vi "ReadRackControllerParameters(BothRacks).vi"(8 "error in":errorcluster, 9 "Part Name":string, 10 "JSON file path":path=path "C:/Users/raakeshs/Desktop/ppts/JSON/Write to JSON String/data/Files/test4.json", 11 "Input ListBox Cluster":T1) -> (0 "error out":errorcluster, 3 "output cluster":T1)   [LabVIEW 2015]
uses:
  ZenGage v3.0 UI.lvclass
  Type Definitions/Edit tolerance settings/Rack Selection.ctl
  Type Definitions/Edit tolerance settings/Edit Tolerance Input.ctl
  <vilib>/Utility/miscctls.llb/LVPoint32TypeDef.ctl
  Type Definitions/Edit tolerance settings/ETL controls.ctl
panel:
  in  "Rack Number":i32
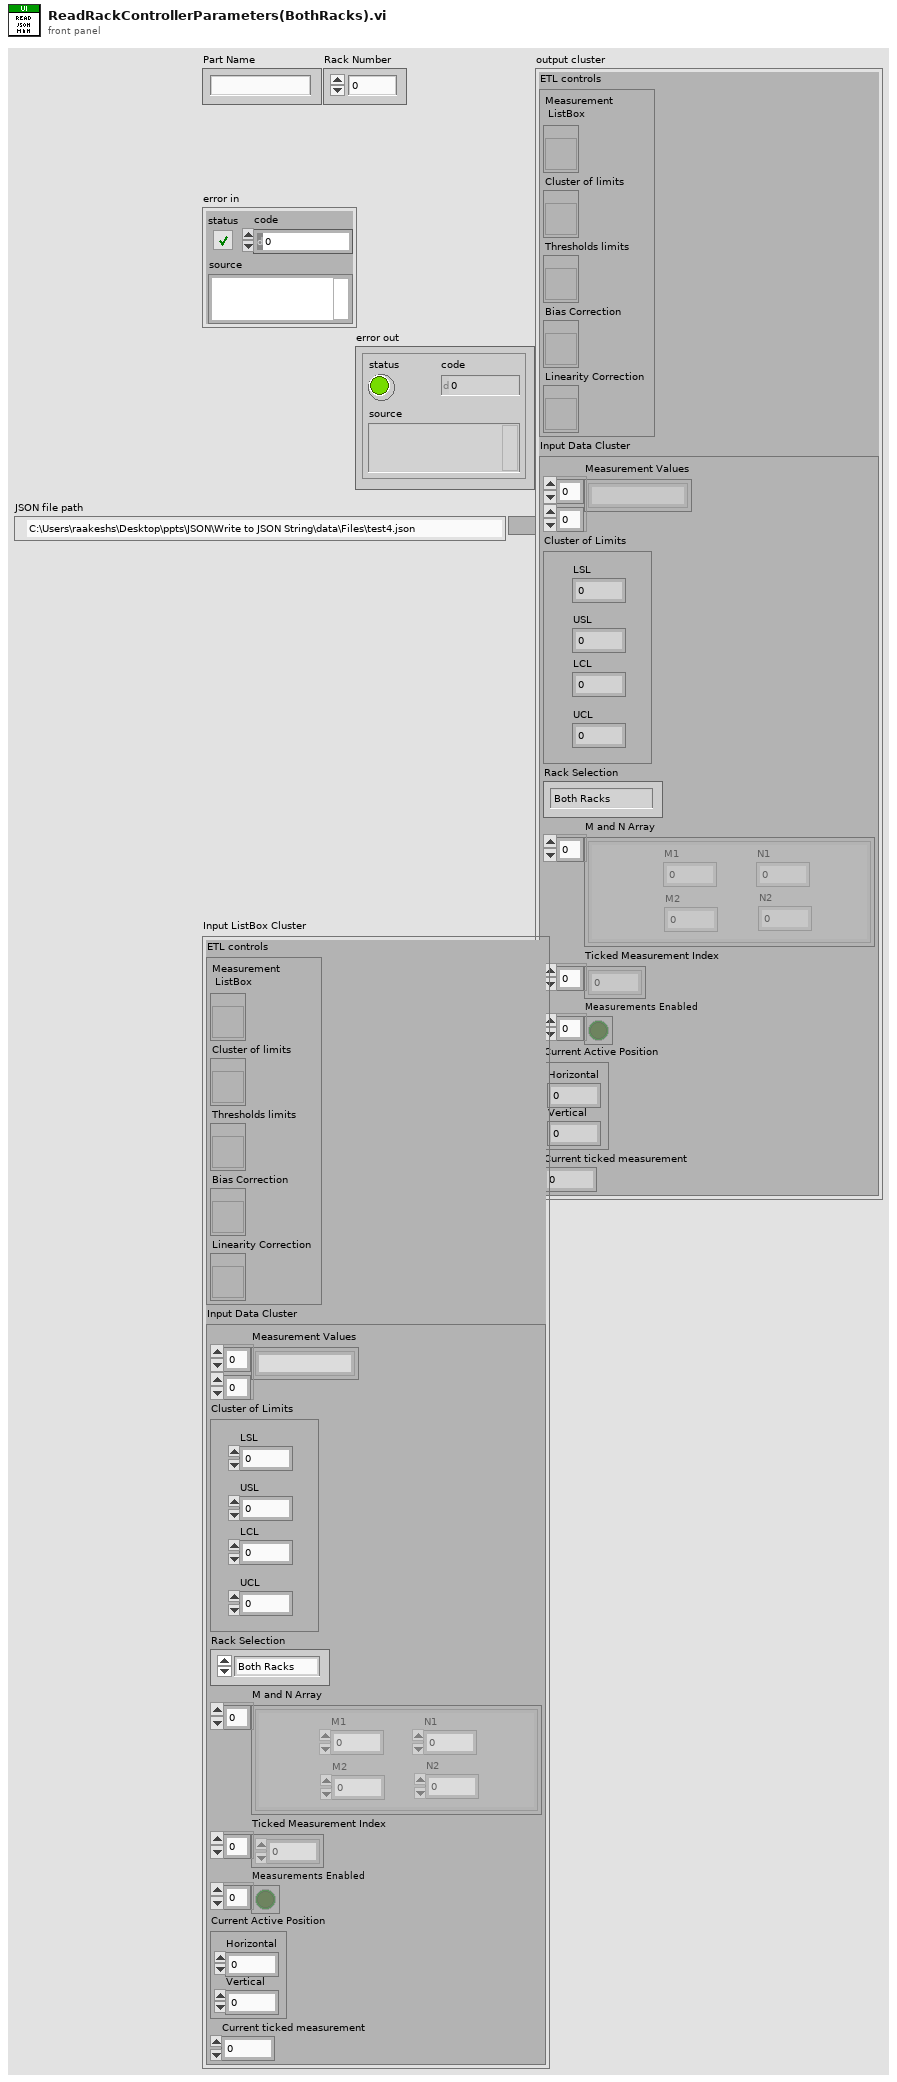
[diagram p1: front panel]
types:
  T1 = typedef "ZenGage v3.0 UI.lvclass/Edit Tolerance Input.ctl" = cluster{"ETL controls":T2, "Input Data Cluster":cluster{"Measurement Values":string[][], "Cluster of Limits":cluster{"LSL":dbl, "USL":dbl, "LCL":dbl, "UCL":dbl}, "Rack Selection":T3, "M and N Array":cluster{"M1":u64, "M2":u64, "N1":u64, "N2":u64}[], "Ticked Measurement Index":u32[], "Measurements Enabled":bool[], "Current Active Position":T4, "Current ticked measurement":dbl}}
  T2 = typedef "ETL controls.ctl" = cluster{"Measurement\n ListBox":refnum<vi>, "Cluster of limits":refnum<vi>, "Thresholds limits":refnum<vi>, "Bias Correction":refnum<vi>, "Linearity Correction":refnum<vi>}
  T3 = typedef "ZenGage v3.0 UI.lvclass/Rack Selection.ctl" = enum16{"Both Racks", "Rack 2", "Rack 1"}
  T4 = typedef "LVPoint32TypeDef.ctl" = cluster{"Horizontal":i32, "Vertical":i32}
  T5 = cluster{"RackControllerParameters":cluster{"RackId":i32, "PartsList":cluster{"Name":string, "ControlLimitsViolationThreshold":cluster{"M1":u64, "N1":u64}, "SpecificationLimitViolationThreshold":cluster{"M2":u64, "N2":u64}}[]}[]}
  T6 = cluster{"RackId":i32, "PartsList":cluster{"Name":string, "ControlLimitsViolationThreshold":cluster{"M1":u64, "N1":u64}, "SpecificationLimitViolationThreshold":cluster{"M2":u64, "N2":u64}}[]}[]
  T7 = cluster{"RackId":i32, "PartsList":cluster{"Name":string, "ControlLimitsViolationThreshold":cluster{"M1":u64, "N1":u64}, "SpecificationLimitViolationThreshold":cluster{"M2":u64, "N2":u64}}[]}
  T8 = cluster{"Name":string, "ControlLimitsViolationThreshold":cluster{"M1":u64, "N1":u64}, "SpecificationLimitViolationThreshold":cluster{"M2":u64, "N2":u64}}[]
  T9 = cluster{"Name":string, "ControlLimitsViolationThreshold":cluster{"M1":u64, "N1":u64}, "SpecificationLimitViolationThreshold":cluster{"M2":u64, "N2":u64}}
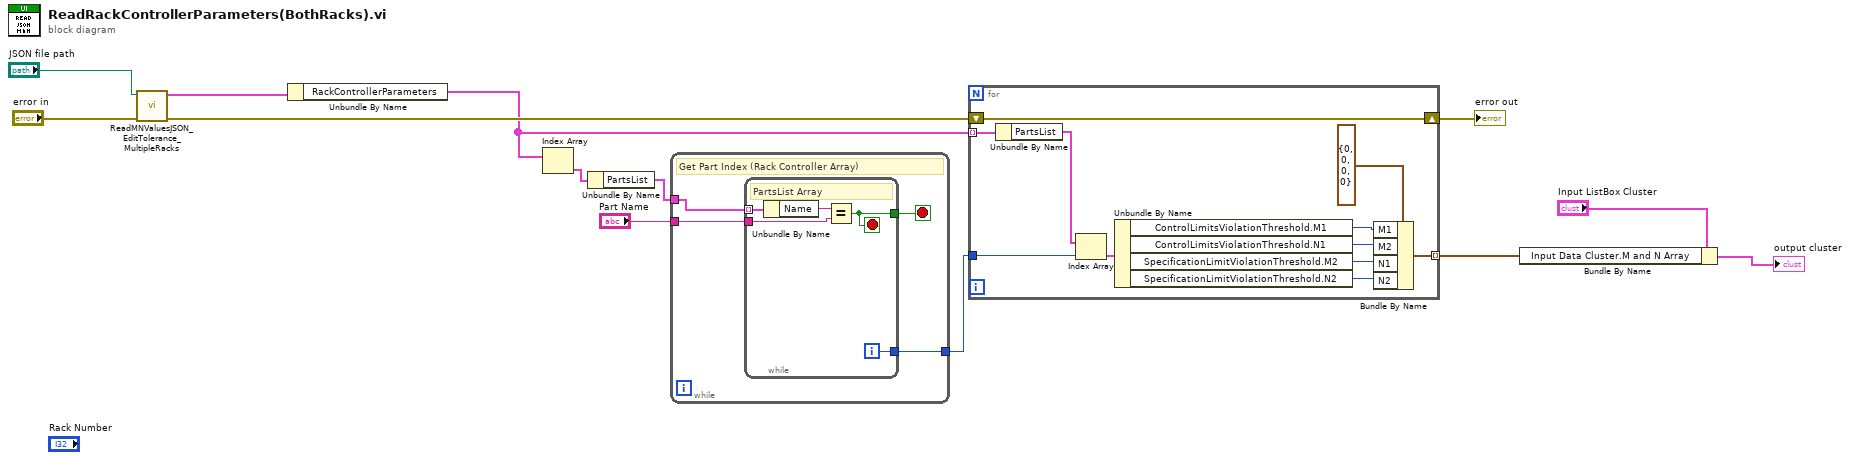
[diagram p0: block diagram]
diagram:
  n1 = call "ReadMNValuesJSON_EditTolerance_MultipleRacks.vi"("error in"="error in", "JSON file path"="JSON file path") -> ("error out"=w10:errorcluster, "Rack Controller Parameters out"=w12:T5)  [unwired: 8 in]
  n2 = Unbundle By Name(w12) -> ("RackControllerParameters"=w7:T6)
  n3 = Index Array(array=w7) -> (element=w2:T7)  [unwired: 1 in]
  n4 = Unbundle By Name(w2) -> ("PartsList"=w1:T8)
  n5 = while {
    tunnel: "Part Name" -> [w17]
    tunnel: [w15] -> w6
    tunnel: w1 -> [w14]
    stop <- w16 stop-if-true
    # "Get Part Index (Rack Controller Array)"
    n6 = while {
      tunnel: w14 -> [w22] mode=indexing
      tunnel: w17 -> [w20]
      tunnel: [w19] -> w16
      tunnel: [w18] -> w15
      i -> [w18]
      stop <- w19 stop-if-true
      # "PartsList Array"
      n7 = Unbundle By Name(w22) -> ("Name"=w21:string)
      n8 = Equal?(x=w21, y=w20) -> (x = y?=w19:bool)
    }
  }
  n9 = for {
    tunnel: w7 -> [w33] mode=indexing
    tunnel: [w32] -> w4 mode=indexing
    shift-right: [w31] -> w9
    shift-left: w10 -> [w31]
    tunnel: w6 -> [w27]
    n10 = Unbundle By Name(w33) -> ("PartsList"=w28:T8)
    n11 = Index Array(array=w28, index=w27) -> (element=w26:T9)
    n12 = Unbundle By Name(w26) -> ("ControlLimitsViolationThreshold.M1"=w30:u64, "ControlLimitsViolationThreshold.N1"=w24:u64, "SpecificationLimitViolationThreshold.M2"=w23:u64, "SpecificationLimitViolationThreshold.N2"=w25:u64)
    n13 = Bundle By Name(cluster=cluster{"M1":u64, "M2":u64, "N1":u64, "N2":u64} {"M1"=0, "M2"=0, "N1"=0, "N2"=0} ("Rack 1"), "M1"=w30, "M2"=w24, "N1"=w23, "N2"=w25) -> (w32:cluster{"M1":u64, "M2":u64, "N1":u64, "N2":u64})
  }
  "error out" <- w9
  n14 = Bundle By Name(cluster="Input ListBox Cluster", "Input Data Cluster.M and N Array"=w4) -> (→"output cluster":T1)
